vi "HumanExecute.vi"(8 "error in (no error)":errorcluster) -> (0 "error out":errorcluster)   [LabVIEW 2020]
doc: "Execute for Human\n\ninput:\n error in (cluster)\n\noutput:\n error out (cluster)"
uses:
  <vilib>/Rock Robotics/WPI/Joystick/XBox Buttons Indexer.ctl
  <vilib>/Rock Robotics/WPI/Joystick/XBox Axes Indexer.ctl
  Arm/ArmGamePiecePreset.ctl
  Arm/ArmPositionPreset.ctl
  Claw/ClawGlobal.vi
  <vilib>/Rock Robotics/WPI/ThirdParty/JAS_Junk/TrajLib/Trajectory_Library.lvlib
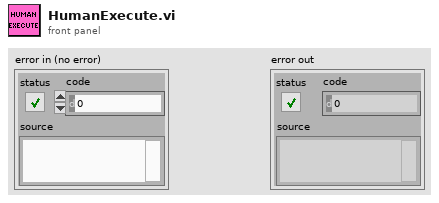
[diagram p1: front panel]
types:
  T1 = typedef "XBox Buttons Indexer.ctl" = enum16{"A", "B", "X", "Y", "Left Bumper", "Right Bumper", "Back", "Start", "Left Joystick", "Right Joystick"}
  T2 = typedef "XBox Axes Indexer.ctl" = enum16{"Left X", "Left Y", "Left Trigger", "Right Trigger", "Right X", "Right Y"}
  T3 = typedef "WPI_JoystickDevRef.ctl" = cluster{"Device":T4}
  T4 = typedef "WPI_JoystickDeviceEnum.ctl" = enum16{"USB 0", "USB 1", "USB 2", "USB 3", "USB 4", "USB 5"}
  T5 = typedef "ArmPositionPreset.ctl" = enum16{"Upper", "Lower", "Middle", "Home", "Shelf", "Floor", "HalfFloor", "HalfHome"}
  T6 = typedef "ArmGamePiecePreset.ctl" = enum16{"Cube", "Cone"}
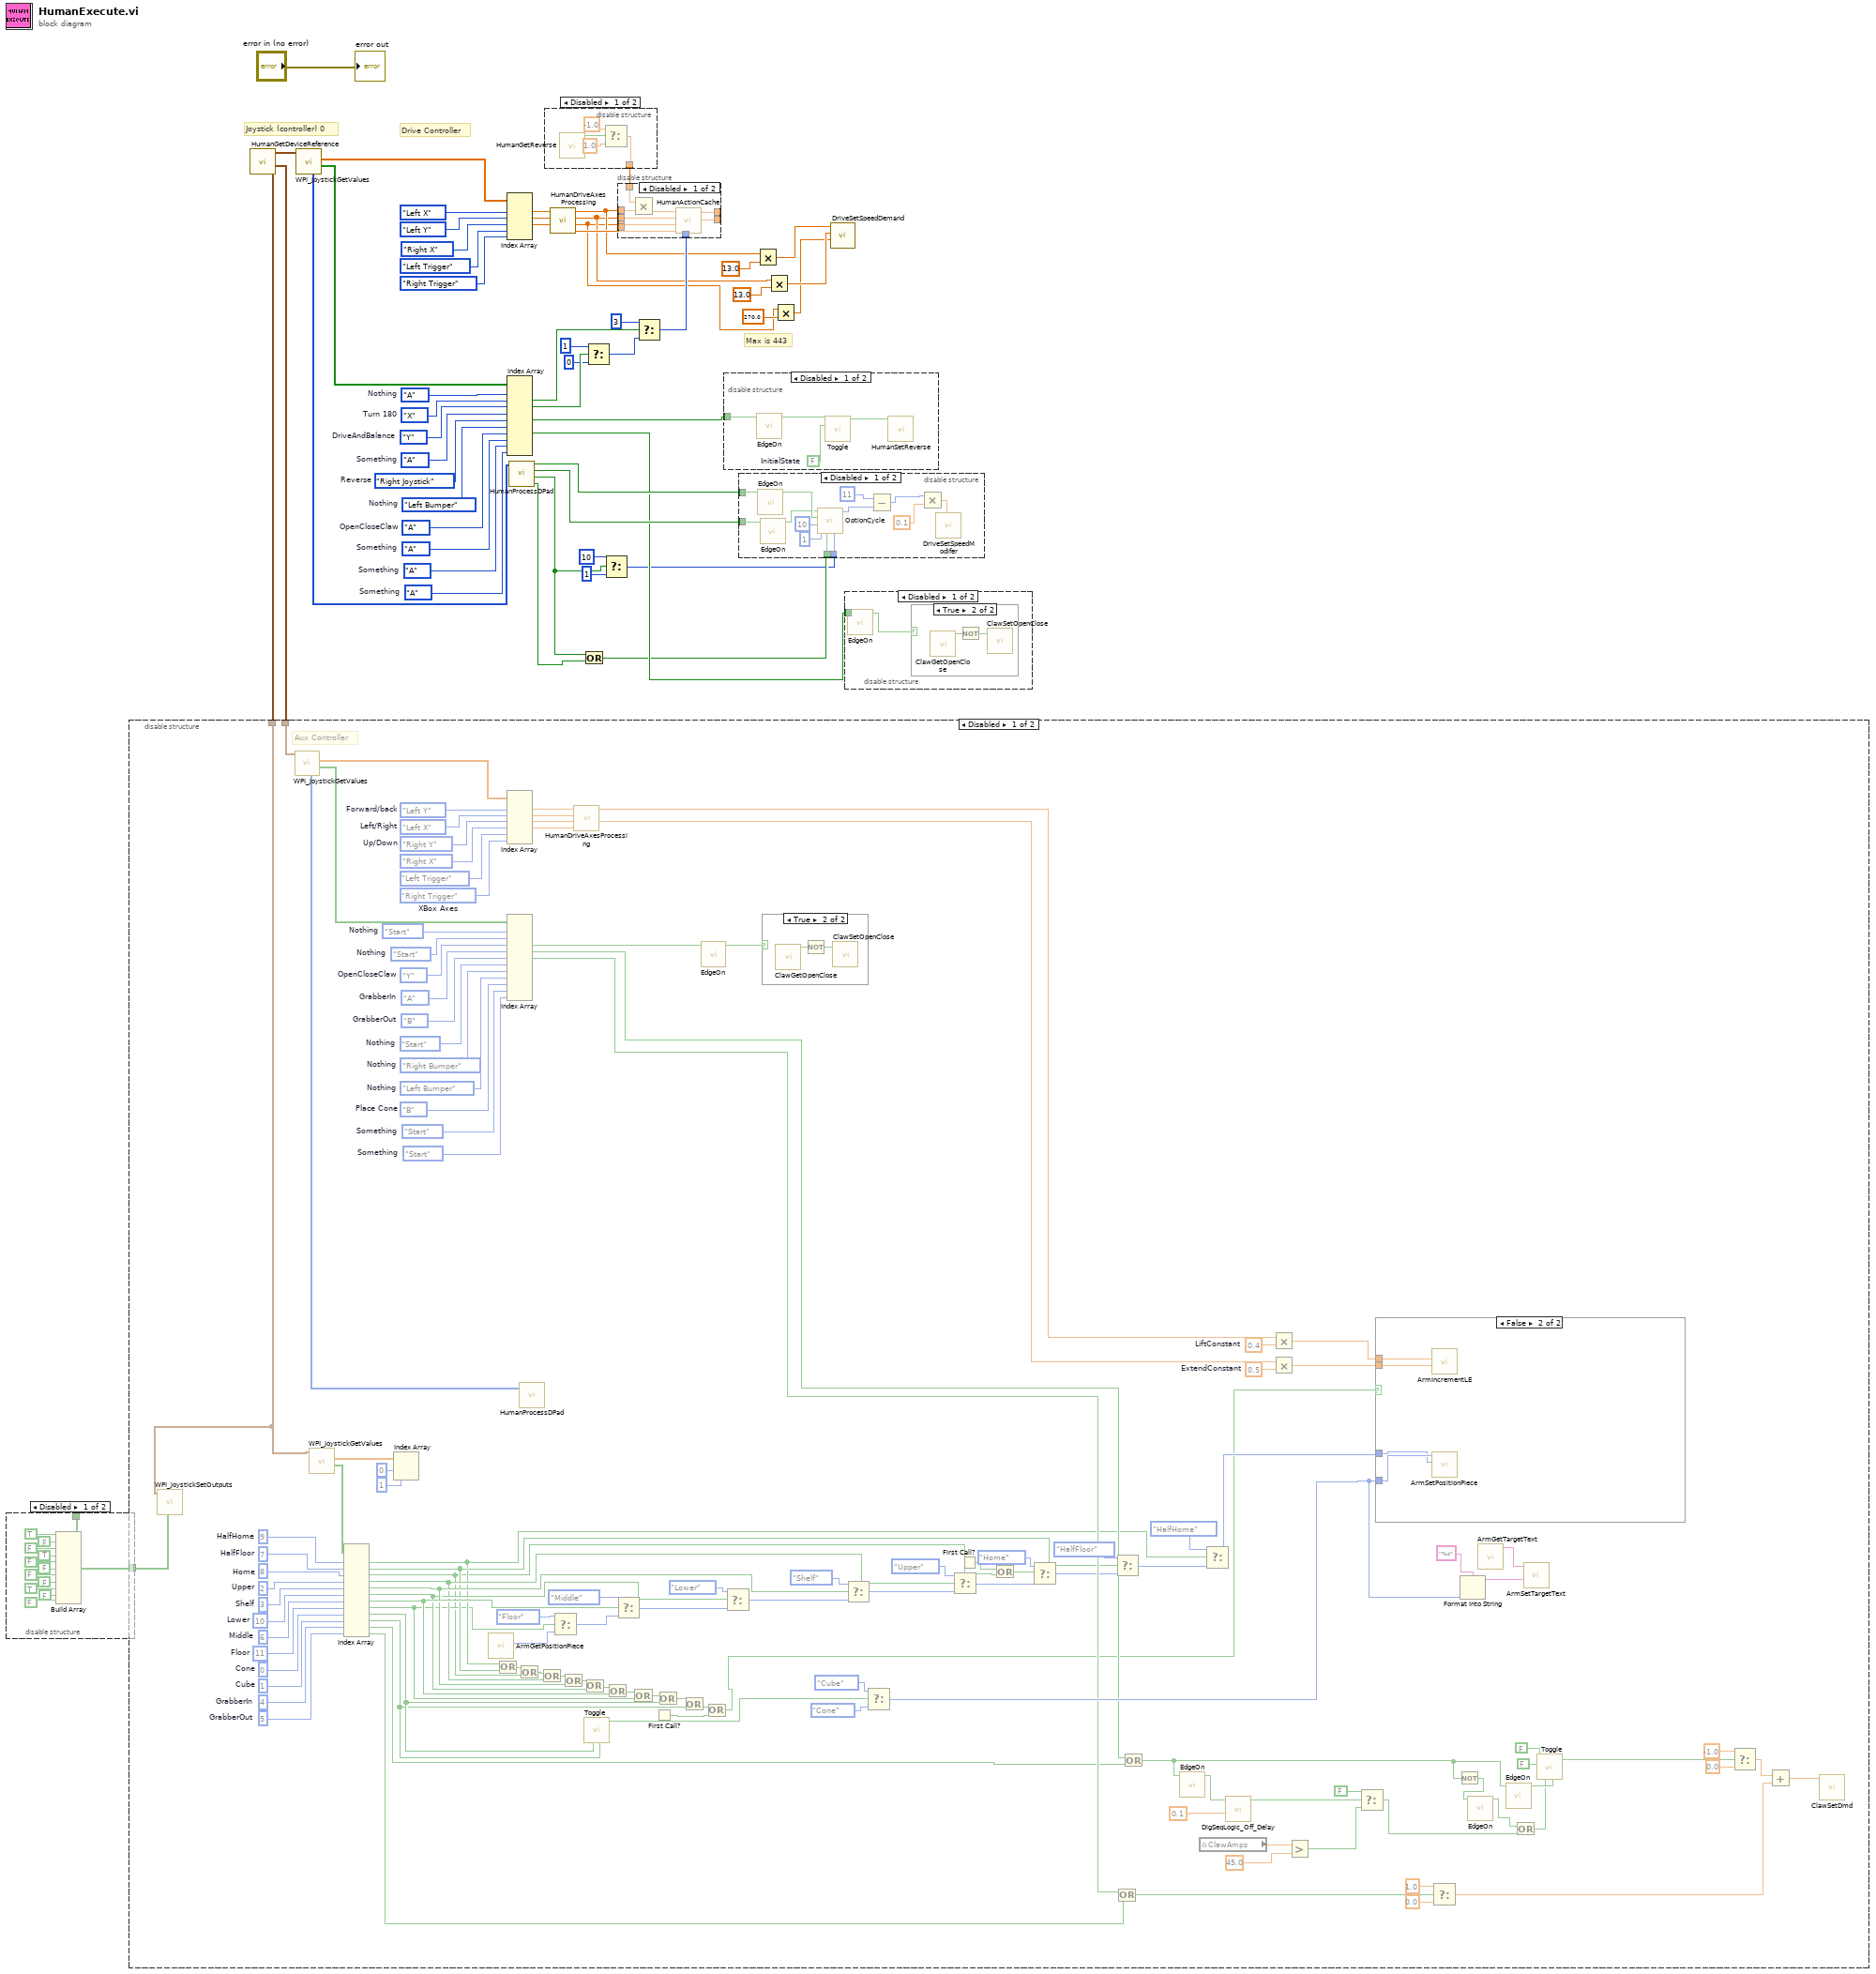
[diagram p0: block diagram]
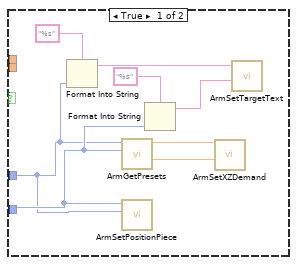
[diagram p9: hidden frame]
diagram:
  w31 = XBox_Buttons_Indexer."A"  # Something
  w32 = XBox_Buttons_Indexer."A"  # Something
  w33 = XBox_Buttons_Indexer."A"  # Something
  w34 = XBox_Buttons_Indexer."A"  # OpenCloseClaw
  w35 = XBox_Buttons_Indexer."Left Bumper"  # Nothing
  w42 = XBox_Buttons_Indexer."Right Joystick"  # Reverse
  w43 = XBox_Buttons_Indexer."A"  # Something
  w45 = XBox_Buttons_Indexer."Y"  # DriveAndBalance
  w46 = XBox_Buttons_Indexer."X"  # Turn 180
  w47 = XBox_Buttons_Indexer."A"  # Nothing
  # "Max is 443"
  # "Joystick (controller) 0"
  # "Drive Controller"
  n1 = disable-structure shown="Disabled" {
    disable-tunnel: [w65 _] -> w23
    frame Disabled {
      n2 = Build Array(TRUE, FALSE ("element"), FALSE ("element"), TRUE ("element"), FALSE ("element"), FALSE ("element"), FALSE ("element"), FALSE ("element"), TRUE ("element"), FALSE ("element"), FALSE ("element")) -> (w65:bool[])
    }
    frame Enabled {
    }
  }
  n3 = call "HumanGetDeviceReference.vi"() -> ("ButtonBoard"=w24:T3, "Aux Joy"=w49:T3, "Driver Joy"=w50:T3)  [unwired: 9 in]
  n4 = disable-structure shown="Disabled" {
    disable-tunnel: w49 -> [w192 _]
    disable-tunnel: w24 -> [w124 _]
    disable-tunnel: w23 -> [w123 _]
    frame Disabled {
      w94 = 9  # HalfHome
      w95 = 7  # HalfFloor
      w134 = 8  # Home
      w141 = 0.4  # LiftConstant
      w142 = 0.5  # ExtendConstant
      w154 = 5  # GrabberOut
      w155 = 4  # GrabberIn
      w156 = 1  # Cube
      w157 = 0  # Cone
      w158 = 11  # Floor
      w159 = 6  # Middle
      w160 = 10  # Lower
      w161 = 3  # Shelf
      w162 = 2  # Upper
      w173 = XBox_Buttons_Indexer."Start"  # Something
      w174 = XBox_Buttons_Indexer."Start"  # Something
      w175 = XBox_Buttons_Indexer."B"  # Place Cone
      w176 = XBox_Buttons_Indexer."Left Bumper"  # Nothing
      w177 = XBox_Buttons_Indexer."Right Bumper"  # Nothing
      w178 = XBox_Buttons_Indexer."Start"  # Nothing
      w183 = XBox_Buttons_Indexer."B"  # GrabberOut
      w186 = XBox_Buttons_Indexer."A"  # GrabberIn
      w187 = XBox_Buttons_Indexer."Y"  # OpenCloseClaw
      w188 = XBox_Buttons_Indexer."Start"  # Nothing
      w189 = XBox_Buttons_Indexer."Start"  # Nothing
      w179 = XBox_Axes_Indexer."Right Trigger"  # XBox Axes
      w182 = XBox_Axes_Indexer."Right Y"  # Up/Down
      w190 = XBox_Axes_Indexer."Left X"  # Left/Right
      w191 = XBox_Axes_Indexer."Left Y"  # Forward/back
      # "Aux Controller"
      n5 = call <vilib>:"WPI_JoystickSetOutputs.vi"("Outputs"=w123, "JoystickDevRef"=w124) -> ()  [unwired: 8 in, 2 out]
      n6 = call <vilib>:"WPI_JoystickGetValues.vi"("JoystickDevRef"=w192) -> ("Buttons"=w184:bool[], "Axes"=w185:dbl[], "POVs"=w172:i16[])  [unwired: 6 in, 2 out]
      n7 = call <vilib>:"WPI_JoystickGetValues.vi"("JoystickDevRef"=w124) -> ("Buttons"=w166:bool[], "Axes"=w165:dbl[])  [unwired: 6 in, 3 out]
      n8 = Index Array "Index Array"(array=w166, index #1=w94, index #2=w95, index #3=w134, index #4=w162, index #5=w161, index #6=w160, index #7=w159, index #8=w158, index #9=w157, index #10=w156, index #11=w155, index #12=w154) -> (element #1=w96:bool, element #2=w97:bool, element #3=w71:bool, element #4=w131:bool, element #5=w146:bool, element #6=w140:bool, element #7=w147:bool, element #8=w91:bool, element #9=w120:bool, element #10=w119:bool, element #11=w89:bool, element #12=w107:bool)
      n9 = Index Array "Index Array"(array=w165, index #1=0 ("index"), index #2=1 ("index")) -> ()  [unwired: 2 out]
      n10 = call "ArmGetPositionPiece.vi"() -> ("Position"=w90:T5)  [unwired: 10 in, 1 out]
      n11 = Or(x=w96, y=w97) -> (x .or. y?=w99:bool)
      n12 = Index Array(array=w185, index #1=w191, index #2=w190, index #3=w182, index #4=XBox_Axes_Indexer."Right X" ("XBox Axes"), index #5=XBox_Axes_Indexer."Left Trigger", index #6=w179) -> (element #1=w171:dbl, element #2=w170:dbl, element #3=w169:dbl, element #4=w168:dbl)  [unwired: 2 out]
      n13 = Index Array "Index Array"(array=w184, index #1=w189, index #2=w188, index #3=w187, index #4=w186, index #5=w183, index #6=w178, index #7=w177, index #8=w176, index #9=w175, index #10=w174, index #11=w173) -> (element #3=w145:bool, element #4=w106:bool, element #5=w105:bool)  [unwired: 8 out]
      n14 = Or(x=w99, y=w71) -> (x .or. y?=w98:bool)
      n15 = call "HumanProcessDPad.vi"("POV"=w172) -> ()  [unwired: 7 in, 4 out]
      n16 = Or(x=w98, y=w131) -> (x .or. y?=w132:bool)
      n17 = Select(t=ArmPositionPreset."Floor" ("Position"), s=w91, f=w90) -> (s? t:f=w93:T5)
      n18 = Or(x=w132, y=w146) -> (x .or. y?=w150:bool)
      n19 = call "HumanDriveAxesProcessing.vi"("Right X"=w168, "Right Y"=w169, "Left X"=w170, "Left Y"=w171) -> ("Right Y"=w143:dbl, "Left Y"=w144:dbl)  [unwired: 4 in, 2 out]
      n20 = Or(x=w150, y=w140) -> (x .or. y?=w149:bool)
      n21 = call "Toggle.vi"("SetTrue"=w119, "SetFalse"=w120) -> ("Toggled"=w137:bool)  [unwired: 9 in]
      n22 = Or(x=w149, y=w147) -> (x .or. y?=w148:bool)
      n23 = Select(t=ArmPositionPreset."Middle" ("Position"), s=w147, f=w93) -> (s? t:f=w152:T5)
      n24 = Or(x=w148, y=w91) -> (x .or. y?=w122:bool)
      n25 = First Call?() -> (First Call?: T/F=w68:bool)
      n26 = Or(x=w122, y=w120) -> (x .or. y?=w121:bool)
      n27 = Or(x=w121, y=w119) -> (x .or. y?=w69:bool)
      n28 = call "EdgeOn.vi"("Current State"=w145) -> ("Edge On Found"=w167:bool)  [unwired: 10 in]
      n29 = Or(x=w69, y=w68) -> (x .or. y?=w67:bool)
      n30 = Select(t=ArmPositionPreset."Lower" ("Position"), s=w140, f=w152) -> (s? t:f=w153:T5)
      n31 = case shown="True" w167 {
        frame False {
        }
        frame True {
          n32 = call "ClawGetOpenClose.vi"() -> ("Open?"=w206:bool)  [unwired: 11 in]
          n33 = Not(x=w206) -> (.not. x?=w205:bool)
          n34 = call "ClawSetOpenClose.vi"("Open?"=w205) -> ()  [unwired: 11 in]
        }
      }
      n35 = Select(t=ArmPositionPreset."Shelf" ("Position"), s=w146, f=w153) -> (s? t:f=w151:T5)
      n36 = Select(t=ArmGamePiecePreset."Cube" ("Game Piece"), s=w137, f=ArmGamePiecePreset."Cone" ("Game Piece")) -> (s? t:f=w125:T6)
      n37 = Select(t=ArmPositionPreset."Upper" ("Position"), s=w131, f=w151) -> (s? t:f=w133:T5)
      n38 = First Call?() -> (First Call?: T/F=w72:bool)
      n39 = Or(x=w72, y=w71) -> (x .or. y?=w70:bool)
      n40 = Select(t=ArmPositionPreset."Home" ("Position"), s=w70, f=w133) -> (s? t:f=w104:T5)
      n41 = Or(x=w105, y=w107) -> (x .or. y?=w108:bool)
      n42 = Select(t=ArmPositionPreset."HalfFloor", s=w97, f=w104) -> (s? t:f=w103:T5)
      n43 = Or(x=w106, y=w89) -> (x .or. y?=w78:bool)
      n44 = call "EdgeOn.vi"("Current State"=w78) -> ("Edge On Found"=w77:bool)  [unwired: 10 in]
      n45 = global read "ClawGlobal.vi" "ClawAmps"() -> (w84:dbl)
      n46 = Select(t=ArmPositionPreset."HalfHome", s=w96, f=w103) -> (s? t:f=w100:T5)
      n47 = call <vilib>:"DigSeqLogic_Off_Delay.vi"("Delay"=0.1 ("Off Delay Tme\nSeconds"), "Input"=w77) -> ("Output"=w76:bool)  [unwired: 8 in, 1 out]
      n48 = Multiply(x=w144, y=w141) -> (x*y=w138:dbl)
      n49 = Multiply(x=w143, y=w142) -> (x*y=w139:dbl)
      n50 = Greater?(x=w84, y=45.0) -> (0:w75:bool)
      n51 = Select(t=FALSE, s=w76, f=w75) -> (s? t:f=w73:bool)
      n52 = case shown="False" w67 {
        tunnel: w139 -> [_ w204]
        tunnel: w138 -> [_ w203]
        tunnel: w125 -> [w194 w202]
        tunnel: w100 -> [w193 w201]
        frame True {
          n53 = Format Into String(format string="%s", w193) -> (resulting string=w198:string)  [unwired: 2 in, 1 out]
          n54 = call "ArmGetPresets.vi"("Game Piece"=w194, "Position"=w193) -> ("z"=w199:dbl, "x"=w200:dbl)  [unwired: 8 in]
          n55 = call "ArmSetPositionPiece.vi"("Position"=w193, "Game Piece"=w194) -> ()  [unwired: 10 in]
          n56 = Format Into String(format string="%s", w194) -> (resulting string=w195:string)  [unwired: 2 in, 1 out]
          n57 = call "ArmSetXZDemand.vi"("SetZ"=w199, "SetX"=w200) -> ()  [unwired: 10 in]
          n58 = call "ArmSetTargetText.vi"("TargetGamePiece"=w195, "TargetArmPosition"=w198) -> ()  [unwired: 10 in]
        }
        frame False {
          n59 = call "ArmIncrementLE.vi"("AddE"=w204, "AddL"=w203) -> ()  [unwired: 10 in]
          n60 = call "ArmSetPositionPiece.vi"("Position"=w201, "Game Piece"=w202) -> ()  [unwired: 10 in]
        }
      }
      n61 = Select(t=1.0, s=w108, f=0.0) -> (s? t:f=w114:dbl)
      n62 = Not(x=w78) -> (.not. x?=w80:bool)
      n63 = Format Into String(format string="%s", w125) -> (resulting string=w118:string)  [unwired: 2 in, 1 out]
      n64 = call "EdgeOn.vi"("Current State"=w80) -> ("Edge On Found"=w81:bool)  [unwired: 10 in]
      n65 = call "ArmGetTargetText.vi"() -> ("TargetArmPosition"=w116:string)  [unwired: 10 in, 1 out]
      n66 = call "EdgeOn.vi"("Current State"=w78) -> ("Edge On Found"=w88:bool)  [unwired: 10 in]
      n67 = Or(x=w81, y=w73) -> (x .or. y?=w82:bool)
      n68 = call "ArmSetTargetText.vi"("TargetGamePiece"=w118, "TargetArmPosition"=w116) -> ()  [unwired: 10 in]
      n69 = call "Toggle.vi"("SetTrue"=w88, "SetFalse"=w82, "InitialState"=FALSE, "FlashInput"=FALSE) -> ("Toggled"=w87:bool)  [unwired: 7 in]
      n70 = Select(t=-1.0, s=w87, f=0.0) -> (s? t:f=w115:dbl)
      n71 = Add(x=w115, y=w114) -> (x+y=w113:dbl)
      n72 = call "ClawSetDmd.vi"("ClawDemand"=w113) -> ()  [unwired: 11 in]
    }
    frame Enabled {
    }
  }
  n73 = call <vilib>:"WPI_JoystickGetValues.vi"("JoystickDevRef"=w50) -> ("Buttons"=w48:bool[], "Axes"=w54:dbl[], "POVs"=w44:i16[])  [unwired: 6 in, 2 out]
  n74 = Index Array(array=w54, index #1=XBox_Axes_Indexer."Left X" ("XBox Axes"), index #2=XBox_Axes_Indexer."Left Y" ("XBox Axes"), index #3=XBox_Axes_Indexer."Right X" ("XBox Axes"), index #4=XBox_Axes_Indexer."Left Trigger" ("XBox Axes"), index #5=XBox_Axes_Indexer."Right Trigger" ("XBox Axes")) -> (element #1=w40:dbl, element #2=w39:dbl, element #3=w38:dbl)  [unwired: 2 out]
  n75 = Index Array(array=w48, index #1=w47, index #2=w46, index #3=w45, index #4=w43, index #5=w42, index #6=w35, index #7=w34, index #8=w33, index #9=w32, index #10=w31) -> (element #2=w14:bool, element #3=w36:bool, element #5=w30:bool, element #7=w25:bool)  [unwired: 6 out]
  n76 = call "HumanProcessDPad.vi"("POV"=w44) -> ("Right"=w21:bool, "Left"=w20:bool, "Down"=w27:bool, "Up"=w28:bool)  [unwired: 7 in]
  n77 = disable-structure shown="Disabled" {
    disable-tunnel: [w207 _] -> w29
    frame Disabled {
      n78 = call "HumanGetReverse.vi"() -> ("Reverse"=w210:bool)  [unwired: 11 in]
      n79 = Select(t=-1.0, s=w210, f=1.0) -> (s? t:f=w207:dbl)
    }
    frame Enabled {
    }
  }
  n80 = call "HumanDriveAxesProcessing.vi"("Right Y"=w38, "Left X"=w39, "Left Y"=w40) -> ("Right X"=w37:dbl, "Right Y"=w1:dbl, "Left X"=w5:dbl, "Left Y"=w9:dbl)  [unwired: 5 in]
  n81 = Or(x=w20, y=w21) -> (x .or. y?=w22:bool)
  n82 = Select(t=1, s=w36, f=0) -> (s? t:f=w15:i32)
  n83 = Select(t=10 ("MinValue"), s=w20, f=1) -> (s? t:f=w17:i32)
  n84 = Select(t=3, s=w14, f=w15) -> (s? t:f=w13:i32)
  n85 = disable-structure shown="Disabled" {
    disable-tunnel: w5 -> [w219 _]
    disable-tunnel: w1 -> [w218 _]
    disable-tunnel: w37 -> [w217 _]
    disable-tunnel: w29 -> [w216 _]
    disable-tunnel: w9 -> [w215 _]
    disable-tunnel: [w213 _] -> _
    disable-tunnel: [w212 _] -> _
    disable-tunnel: w13 -> [w211 _]
    frame Disabled {
      n86 = Multiply(x=w216, y=w215) -> (x*y=w214:dbl)
      n87 = call "HumanActionCache.vi"("State"=w211, "Right X"=w217, "Right Y"=w218, "Left X"=w219, "Left Y"=w214) -> ("RightMotorDemand"=w212:dbl, "LeftMotorDemand"=w213:dbl)  [unwired: 5 in]
    }
    frame Enabled {
    }
  }
  n88 = disable-structure shown="Disabled" {
    disable-tunnel: w30 -> [w221 _]
    frame Disabled {
      w222 = FALSE  # InitialState
      n89 = call "EdgeOn.vi"("Current State"=w221) -> ("Edge On Found"=w223:bool)  [unwired: 10 in]
      n90 = call "Toggle.vi"("InitialState"=w222, "FlashInput"=w223) -> ("Toggled"=w220:bool)  [unwired: 9 in]
      n91 = call "HumanSetReverse.vi"("Reverse"=w220) -> ()  [unwired: 11 in]
    }
    frame Enabled {
    }
  }
  n92 = disable-structure shown="Disabled" {
    disable-tunnel: w28 -> [w231 _]
    disable-tunnel: w27 -> [w230 _]
    disable-tunnel: w22 -> [w225 _]
    disable-tunnel: w17 -> [w224 _]
    frame Disabled {
      n93 = call "EdgeOn.vi"("Current State"=w231) -> ("Edge On Found"=w229:bool)  [unwired: 10 in]
      n94 = call "EdgeOn.vi"("Current State"=w230) -> ("Edge On Found"=w228:bool)  [unwired: 10 in]
      n95 = call "OptionCycle.vi"("ValuetoSet"=w224, "SetValue"=w225, "MinValue"=1, "MaxValue"=10, "BackwardsInput"=w229, "ForwardInput"=w228) -> ("CycleNum"=w234:i32)  [unwired: 5 in]
      n96 = Subtract(x=11, y=w234) -> (x-y=w232:i32)
      n97 = Multiply(x=w232, y=0.1) -> (x*y=w235:dbl)
      n98 = call "DriveSetSpeedModifer.vi"("SpeedModifer"=w235) -> ()  [unwired: 11 in]
    }
    frame Enabled {
    }
  }
  n99 = Multiply(x=w9, y=13.0) -> (x*y=w7:dbl)
  n100 = Multiply(x=w5, y=13.0) -> (x*y=w4:dbl)
  n101 = Multiply(x=w1, y=270.0) -> (x*y=w2:dbl)
  n102 = call "DriveSetSpeedDemand.vi"("ASpeedDemand (d/s)"=w2, "YSpeedDemand (ft/s)"=w4, "XSpeedDemand (ft/s)"=w7) -> ()  [unwired: 9 in]
  n103 = disable-structure shown="Disabled" {
    disable-tunnel: w25 -> [w238 _]
    frame Disabled {
      n104 = call "EdgeOn.vi"("Current State"=w238) -> ("Edge On Found"=w237:bool)  [unwired: 10 in]
      n105 = case shown="True" w237 {
        frame False {
        }
        frame True {
          n106 = call "ClawGetOpenClose.vi"() -> ("Open?"=w240:bool)  [unwired: 11 in]
          n107 = Not(x=w240) -> (.not. x?=w239:bool)
          n108 = call "ClawSetOpenClose.vi"("Open?"=w239) -> ()  [unwired: 11 in]
        }
      }
    }
    frame Enabled {
    }
  }
  "error out" <- "error in (no error)"
